vi "Set REF f equal AO f.vi"(10 "REE = AO?":bool, 11 "Cluster in":T1) -> (3 "Cluster out 2":T1)   [LabVIEW 2013]
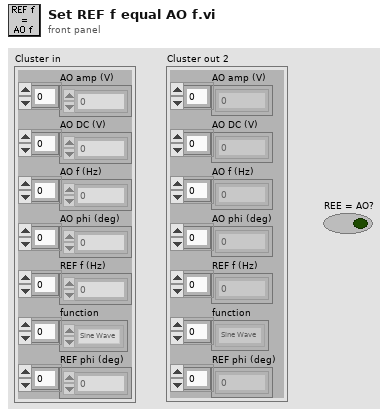
[diagram p1: front panel]
types:
  T1 = cluster{"AO amp (V)":dbl[], "AO DC (V)":dbl[], "AO f (Hz)":dbl[], "AO phi (deg)":dbl[], "REF f (Hz)":dbl[], "function":enum16{"Sine Wave", "Triangle Wave", "Square Wave", "Sawtooth Wave"}[], "REF phi (deg)":dbl[]}
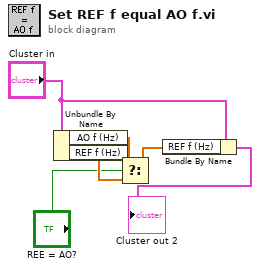
[diagram p0: block diagram]
diagram:
  n1 = Unbundle By Name("Cluster in") -> ("AO f (Hz)"=w2:dbl[], "REF f (Hz)"=w4:dbl[])
  n2 = Select(t=w2, s="REE = AO?", f=w4) -> (s? t:f=w3:dbl[])
  n3 = Bundle By Name(cluster="Cluster in", "REF f (Hz)"=w3) -> (→"Cluster out 2":T1)
